vi "Read Pigeon.vi"(11 "PigeonIMUDevRef":T1 {"Type" items=["CAN"=352321536, "TalonSRX"=33554432]}) -> (2 "Yaw":dbl)   [LabVIEW 2018]
uses:
  <vilib>/Rock Robotics/WPI/ThirdParty/Phoenix-LabVIEW/Pigeon IMU/CTRE_PigeonIMU_DeviceRef.ctl
  <vilib>/Rock Robotics/WPI/ThirdParty/Phoenix-LabVIEW/Pigeon IMU/CTRE_PigeonIMU_ConnectionType.ctl
  <vilib>/Rock Robotics/WPI/ThirdParty/Phoenix-LabVIEW/Pigeon IMU/CTRE_PigeonIMU_GetYPR.vi
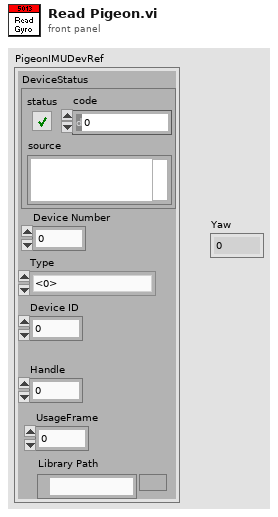
[diagram p1: front panel]
types:
  T1 = typedef "CTRE_PigeonIMU_DeviceRef.ctl" = cluster{"DeviceStatus":errorcluster, "Device Number":u8, "Type":T2, "Device ID":u32, "Handle":u64, "UsageFrame":u32, "Library Path":path}
  T2 = typedef "CTRE_PigeonIMU_ConnectionType.ctl" = u32
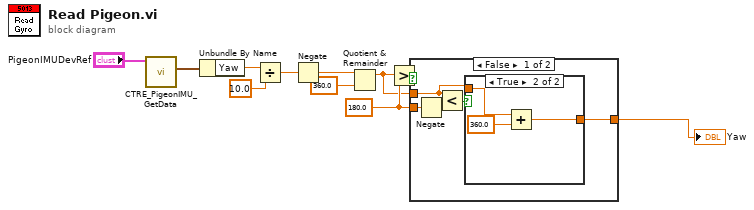
[diagram p0: block diagram]
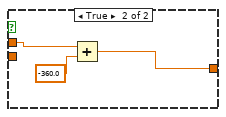
[diagram p3: hidden frame]
diagram:
  w11 = 180.0 ("y")
  n1 = call-poly <vilib>:"CTRE_PigeonIMU_GetData.vi"("PigeonIMUDevRef"="PigeonIMUDevRef") -> ("Yaw Pitch Roll"=w5:cluster{"Yaw":dbl, "Pitch":dbl, "Roll":dbl})  [unwired: 8 in, 2 out]
  n2 = Unbundle By Name(w5) -> ("Yaw"=w7:dbl)
  n3 = Divide(x=w7, y=10.0) -> (x/y=w2:dbl)
  n4 = Negate(x=w2) -> (-x=w3:dbl)
  n5 = Quotient & Remainder(x=w3, y=360.0) -> (x-y*floor(x/y)=w10:dbl)  [unwired: 1 out]
  n6 = Greater?(x=w10, y=w11) -> (0:w9:bool)
  n7 = case shown="False" w9 {
    tunnel: w10 -> [w14 w22]
    tunnel: w11 -> [w13 _]
    tunnel: [w12 w21] -> w4
    frame False {
      n8 = Negate(x=w13) -> (-x=w15:dbl)
      n9 = Less?(x=w14, y=w15) -> (x < y?=w16:bool)
      n10 = case shown="True" w16 {
        tunnel: w14 -> [w17 w20]
        tunnel: [w17 w18] -> w12
        frame False {
        }
        frame True {
          n11 = Add(x=w20, y=360.0) -> (x+y=w18:dbl)
        }
      }
    }
    frame True {
      n12 = Add(x=w22, y=-360.0) -> (x+y=w21:dbl)
    }
  }
  "Yaw" <- w4
